vi "002 Comparador.vi"() -> ()   [LabVIEW 2019]
panel:
  out "A < B":bool
  out "A = B":bool
  out "A > B":bool
  in  "Nombre B":dbl
  in  "Nombre A":dbl
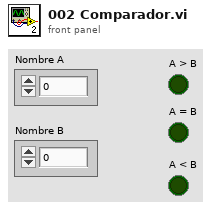
[diagram p1: front panel]
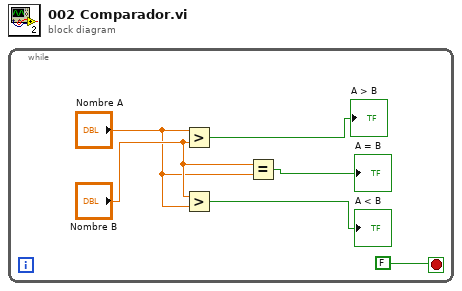
[diagram p0: block diagram]
diagram:
  n1 = while {
    stop <- FALSE stop-if-true
    n2 = Greater?(x="Nombre A", y="Nombre B") -> (0:→"A > B":bool)
    n3 = Greater?(x="Nombre B", y="Nombre A") -> (0:→"A < B":bool)
    n4 = Equal?(x="Nombre B", y="Nombre A") -> (x = y?=→"A = B":bool)
  }
